vi "Initialize SP.vi"(8 "error in (no error)":errorcluster, 11 "subpanel (abstract) in":refnum<class "subpanel (abstract).lvclass">) -> (0 "error out":errorcluster, 3 "subpanel (abstract) out":refnum<class "subpanel (abstract).lvclass">)   [LabVIEW 2023, in "GUI.lvlib" / "subpanel (abstract).lvclass"]
uses:
  subpanel (abstract).lvclass
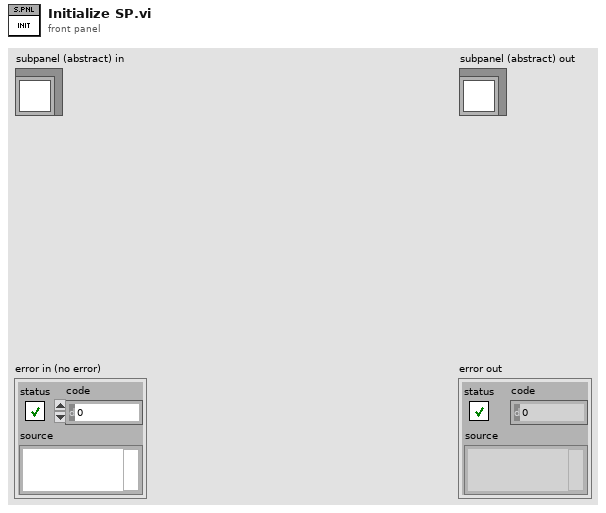
[diagram p1: front panel]
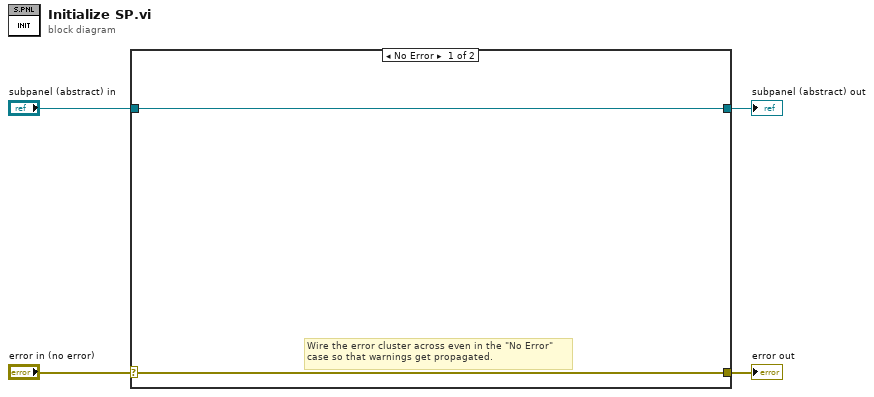
[diagram p0: block diagram]
diagram:
  n1 = case shown="No Error" "error in (no error)" {
    selector: "error in (no error)" -> [w5 w8]
    tunnel: [w5 w8] -> w3
    tunnel: [w6 w7] -> w1
    tunnel: "subpanel (abstract) in" -> [w6 w7]
    frame No Error {
      # "Wire the error cluster across even in the \"No Error\"\ncase so that warnings get propagated."
    }
    frame Error {
    }
  }
  "error out" <- w3
  "subpanel (abstract) out" <- w1
